vi "check internet access (http).vi"(8 "error in (no error)":errorcluster, 11 "timeout (ms)":i32=5000) -> (0 "error out":errorcluster)   [LabVIEW 2016]
uses:
  <vilib>/httpClient/LabVIEWHTTPClient.lvlib
panel:
  out "value":T1
  out "stop scanoutput":string
  out "data out  from LIDAR":string
  in  "Stop Button":bool
  out "start scanoutput":string
  out "error_code":i32
  out "error_text":string
  out "handle":string
  out "body":string
  out "headers":string
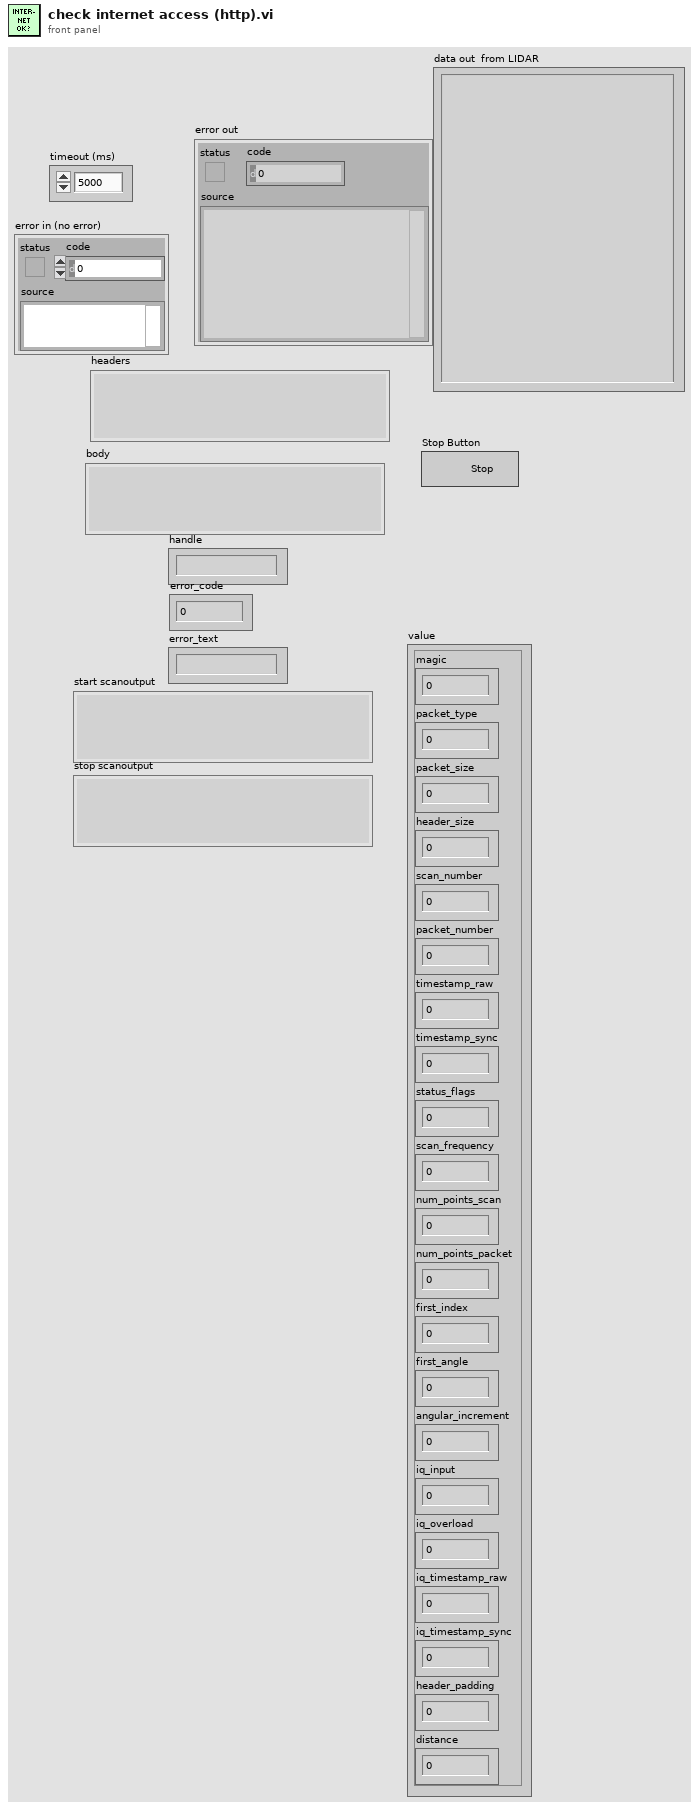
[diagram p1: front panel]
types:
  T1 = cluster{"magic":u16, "packet_type":u16, "packet_size":u32, "header_size":u16, "scan_number":u16, "packet_number":u16, "timestamp_raw":u64, "timestamp_sync":u64, "status_flags":u32, "scan_frequency":u32, "num_points_scan":u16, "num_points_packet":u16, "first_index":u16, "first_angle":i32, "angular_increment":i32, "iq_input":u32, "iq_overload":u32, "iq_timestamp_raw":u64, "iq_timestamp_sync":u64, "header_padding":u8, "distance":u32}
  T2 = cluster{"handle":string, "error_code":i32, "error_text":string}
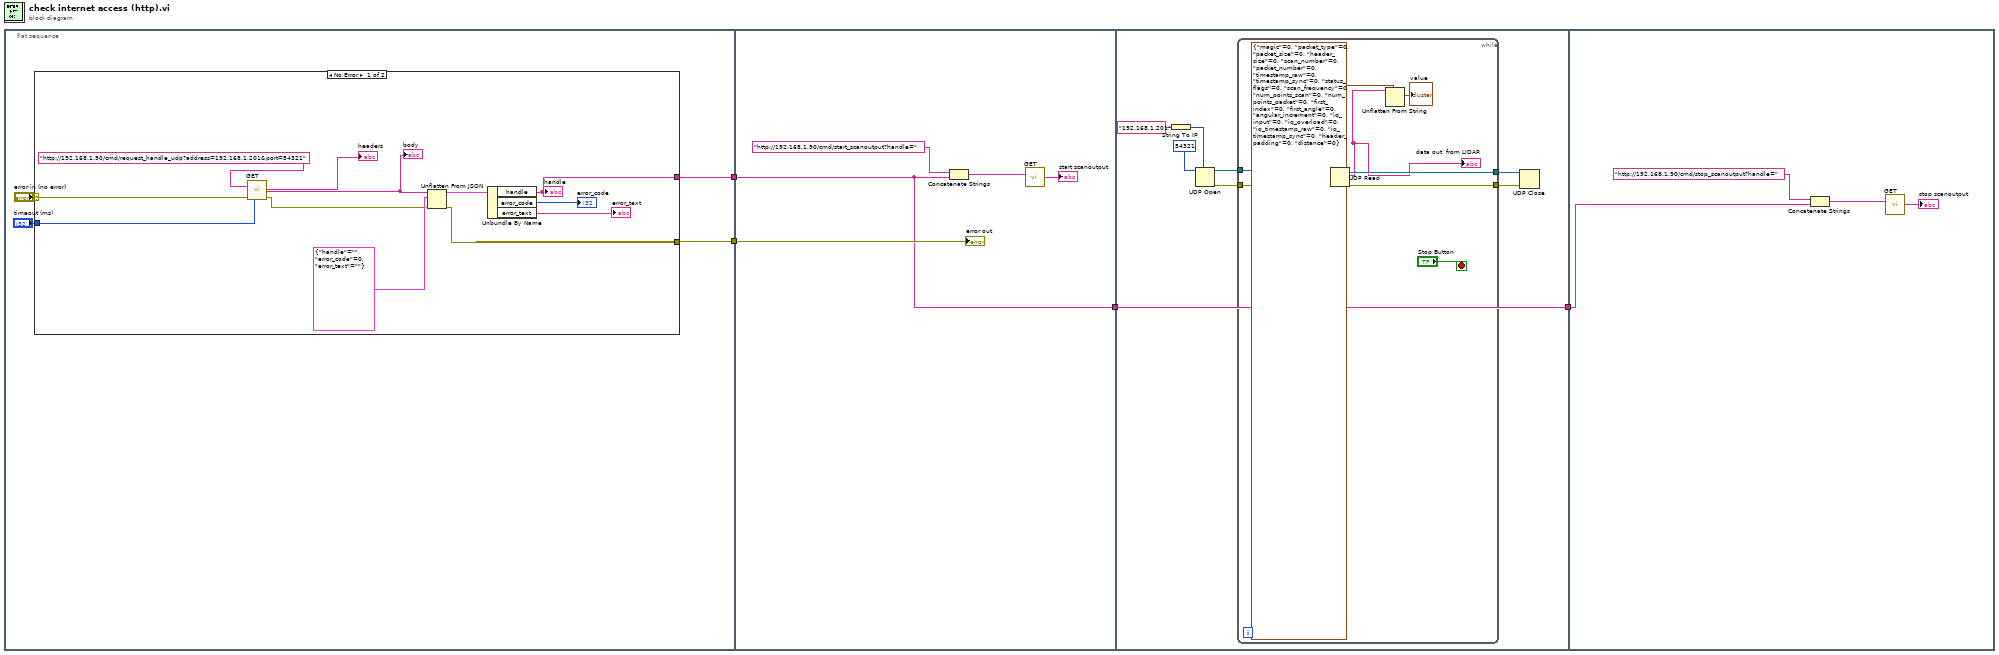
[diagram p0: block diagram]
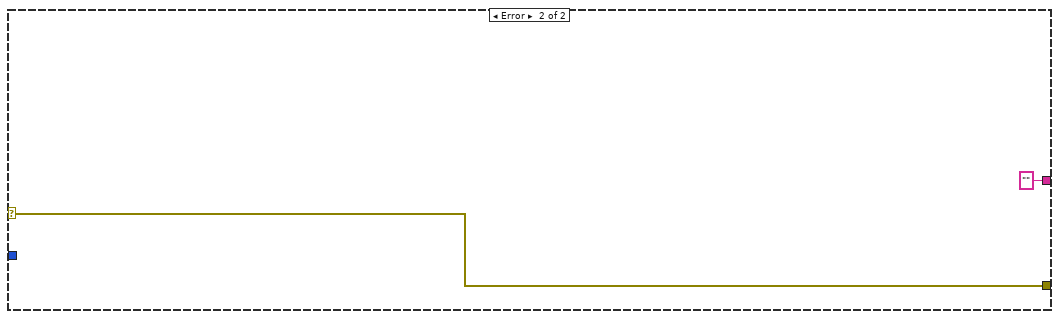
[diagram p2: hidden frame]
diagram:
  n1 = flat-sequence {
    tunnel: [w6] -> w4
    tunnel: [w5] -> w3
    tunnel: w4 -> [w23]
    tunnel: w3 -> [w26]
    tunnel: [w23] -> w2
    tunnel: w2 -> [w28]
    tunnel: [w28] -> w1
    tunnel: w1 -> [w44]
    frame #0 {
      n2 = case shown="No Error" "error in (no error)" {
        selector: "error in (no error)" -> [w19 w22]
        tunnel: [w13 w22] -> w5
        tunnel: "timeout (ms)" -> [w18 _]
        tunnel: [w9 "" ("handle")] -> w6
        frame No Error {
          n3 = call <vilib>:"GET.vi"("url"="http://192.168.1.90/cmd/request_handle_udp?address=192.168.1.201&port=54321" ("address"), "error in (no error)"=w19, "timeout (10000)"=w18) -> ("headers"=→"headers":string, "body"=w16:string, "error out"=w14:errorcluster)  [unwired: 9 in, 1 out]
          "body" <- w16
          n4 = Unflatten From JSON(JSON string=w16, type and defaults=T2 {"handle"="", "error_code"=0, "error_text"=""}, error in (no error)=w14) -> (value=w12:T2, error out=w13:errorcluster)  [unwired: 4 in]
          n5 = Unbundle By Name(w12) -> ("handle"=w9:string, "error_code"=→"error_code":i32, "error_text"=→"error_text":string)
          "handle" <- w9
        }
        frame Error {
        }
      }
    }
    frame #1 {
      n6 = Concatenate Strings "Concatenate Strings"("http://192.168.1.90/cmd/start_scanoutput?handle=", w23) -> (w25:string)
      n7 = call <vilib>:"GET.vi"("url"=w25) -> ("body"=→"start scanoutput":string)  [unwired: 11 in, 3 out]
      "error out" <- w26
    }
    frame #2 {
      n8 = String To IP(1:"192.168.1.201" ("name")) -> (0:w34:u32)
      n9 = UDP Open(7:w34, 11:u16 54321 ("port")) -> (port=w32:refnum<k16>, 0:w31:errorcluster)  [unwired: 3 in, 1 out]
      n10 = while {
        tunnel: w32 -> [w42]
        tunnel: w31 -> [w41]
        tunnel: [w40] -> w30
        tunnel: [w39] -> w29
        stop <- "Stop Button" stop-if-true
        n11 = UDP Read(connection ID=w42, 8:w41) -> (data out=w38:string, error out=w40:errorcluster, 3:w39:refnum<k16>)  [unwired: 2 in, 2 out]
        "data out  from LIDAR" <- w38
        n12 = Unflatten From String(type=T1 {"magic"=0, "packet_type"=0, "packet_size"=0, "header_size"=0, "scan_number"=0, "packet_number"=0, "timestamp_raw"=0, "timestamp_sync"=0, "status_flags"=0, "scan_frequency"=0, "num_points_scan"=0, "num_points_packet"=0, "first_index"=0, "first_angle"=0, "angular_increment"=0, "iq_input"=0, "iq_overload"=0, "iq_timestamp_raw"=0, "iq_timestamp_sync"=0, "header_padding"=0, "distance"=0}, binary string=w38) -> (value=→"value":T1)  [unwired: 3 in, 2 out]
      }
      n13 = UDP Close(connection ID=w29, 8:w30) -> ()  [unwired: 2 out]
    }
    frame #3 {
      n14 = Concatenate Strings "Concatenate Strings"("http://192.168.1.90/cmd/stop_scanoutput?handle=", w44) -> (w46:string)
      n15 = call <vilib>:"GET.vi"("url"=w46) -> ("body"=→"stop scanoutput":string)  [unwired: 11 in, 3 out]
    }
  }
